vi "Z900_navX_Util_BigEndian_to_LittleEndian.vi"(1 "Big Endian":u8[](array[numeric])) -> (0 "Little Endian":u8[](array[numeric]))   [LabVIEW 2016, in "navX Library.lvlib"]
uses:
  navX Library.lvlib
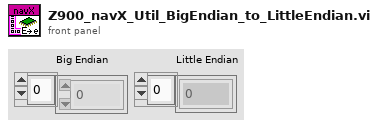
[diagram p1: front panel]
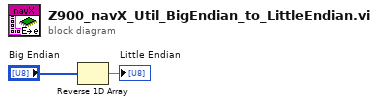
[diagram p0: block diagram]
diagram:
  n1 = Reverse 1D Array(array="Big Endian") -> (reversed array=→"Little Endian":u8[])
